vi "Deco meds ME.vi"(5 "Eeprom":T2 {"Analogicas 32"."?" items=["1", "2", "4", "8", "16", "32", "64", "128", "256"]; "Analogicas 32"."?" items=["Lineal"=15, "Cuadrática"=14]; "Analogicas 32"."unsigned byte array[0]" items=["10000", "1000", "100", "10", "8000", "800", "80", "8", "4000", "400", "40", "4", "2000", "200", "20", "2"]; "Analogicas 16"."?" items=["1", "2", "4", "8", "16", "32", "64", "128", "256"]; "Analogicas 16"."?" items=["Lineal"=15, "Cuadrática"=14]; "Analogicas 16"."unsigned byte array[0]" items=["10000", "1000", "100", "10", "8000", "800", "80", "8", "4000", "400", "40", "4", "2000", "200", "20", "2"]}, 6 "data IN":string) -> (3 "Med 568":T1)   [LabVIEW 2010]
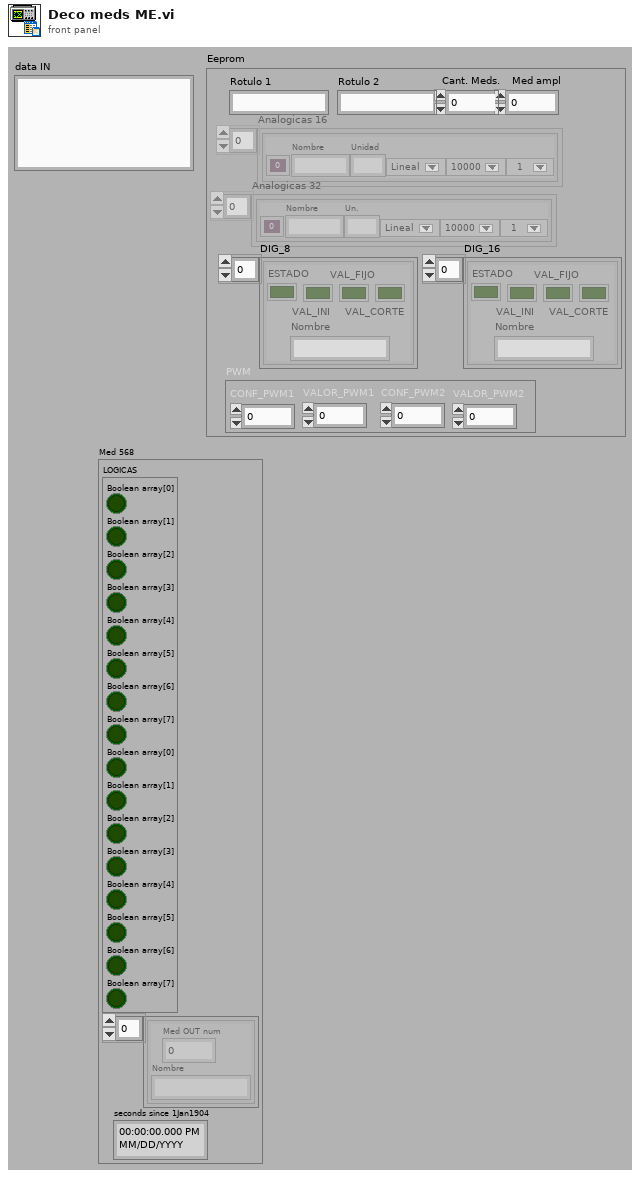
[diagram p1: front panel]
types:
  T1 = cluster{"LOGICAS":cluster{"Boolean array[0]":bool, "Boolean array[1]":bool, "Boolean array[2]":bool, "Boolean array[3]":bool, "Boolean array[4]":bool, "Boolean array[5]":bool, "Boolean array[6]":bool, "Boolean array[7]":bool, "Boolean array[0]":bool, "Boolean array[1]":bool, "Boolean array[2]":bool, "Boolean array[3]":bool, "Boolean array[4]":bool, "Boolean array[5]":bool, "Boolean array[6]":bool, "Boolean array[7]":bool}, cluster{"Med OUT num":dbl, "Nombre":string}[], "seconds since 1Jan1904":timestamp}
  T2 = cluster{"Rotulo 1":string, "Rotulo 2":string, "Cant. Meds.":u8, "Med ampl":u8, "Analogicas 16":cluster{"Nº":i32, "Nombre":string, "Unidad":string, u8, "unsigned byte array[0]":u8, u8}[], "Analogicas 32":cluster{i32, "Nombre":string, "Un.":string, u8, "unsigned byte array[0]":u8, u8}[], "DIG_8":cluster{"ESTADO":bool, "VAL_INI":bool, "VAL_FIJO":bool, "VAL_CORTE":bool, "Nombre":string}[], "DIG_16":cluster{"ESTADO":bool, "VAL_INI":bool, "VAL_FIJO":bool, "VAL_CORTE":bool, "Nombre":string}[], "PWM":cluster{"CONF_PWM1":u8, "VALOR_PWM1":u8, "CONF_PWM2":u8, "VALOR_PWM2":u8}}
  T3 = cluster{"Boolean array[0]":bool, "Boolean array[1]":bool, "Boolean array[2]":bool, "Boolean array[3]":bool, "Boolean array[4]":bool, "Boolean array[5]":bool, "Boolean array[6]":bool, "Boolean array[7]":bool, "Boolean array[0]":bool, "Boolean array[1]":bool, "Boolean array[2]":bool, "Boolean array[3]":bool, "Boolean array[4]":bool, "Boolean array[5]":bool, "Boolean array[6]":bool, "Boolean array[7]":bool}
  T4 = cluster{"Nº":i32, "Nombre":string, "Unidad":string, u8, "unsigned byte array[0]":u8, u8}[]
  T5 = cluster{i32, "Nombre":string, "Un.":string, u8, "unsigned byte array[0]":u8, u8}[]
  T6 = cluster{"Nº":i32, "Nombre":string, "Un.":string, u8, "unsigned byte array[0]":u8, u8}
  T7 = cluster{"LOGICAS":cluster{"Boolean array[0]":bool, "Boolean array[1]":bool, "Boolean array[2]":bool, "Boolean array[3]":bool, "Boolean array[4]":bool, "Boolean array[5]":bool, "Boolean array[6]":bool, "Boolean array[7]":bool, "Boolean array[0]":bool, "Boolean array[1]":bool, "Boolean array[2]":bool, "Boolean array[3]":bool, "Boolean array[4]":bool, "Boolean array[5]":bool, "Boolean array[6]":bool, "Boolean array[7]":bool}, cluster{"Med OUT num":dbl, string}[], "seconds since 1Jan1904":timestamp}
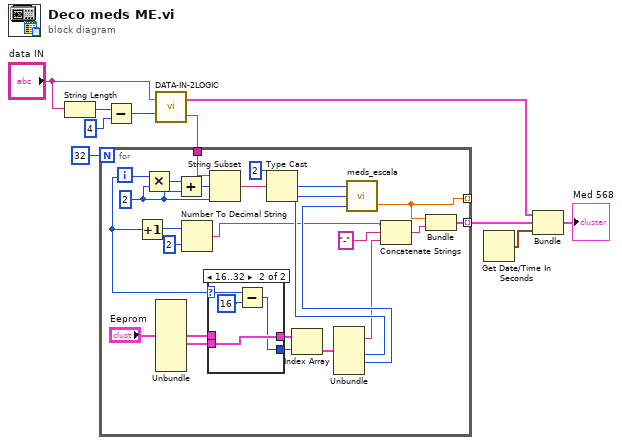
[diagram p0: block diagram]
diagram:
  n1 = String Length(string="data IN") -> (length=w9:i32)
  n2 = Subtract(x=w9, y=4) -> (x-y=w8:i32)
  n3 = call "DATA-IN-2LOGIC.vi"("SIZE"=w8, "data IN"="data IN") -> ("ANALOGICAS"=w5:string, "LOGICAS"=w3:T3)
  n4 = for {
    N: 32 -> [_]
    tunnel: w5 -> [w21]
    tunnel: [w19] -> _ mode=indexing
    tunnel: [w18] -> w2 mode=indexing
    i -> [w17]
    w33 = 2 ("offset (0)")
    n5 = Increment(x=w17) -> (x+1=w16:i32)
    n6 = Multiply(x=w17, y=w33) -> (x*y=w34:i32)
    n7 = Unbundle("Eeprom") -> ("Analogicas 16"=w30:T4, "Analogicas 32"=w29:T5)  [unwired: 7 out]
    n8 = Add(x=w34, y=w33) -> (x+y=w20:i32)
    n9 = Number To Decimal String(number=w16, width (-)=i16 2) -> (decimal integer string=w11:string)
    n10 = case shown="16..32" w17 {
      selector: w17 -> [w35 w40]
      tunnel: w30 -> [w36 _]
      tunnel: w29 -> [_ w38]
      tunnel: [w36 w38] -> w28
      tunnel: [w35 w37] -> w27
      frame 0..15, Default {
      }
      frame 16..32 {
        n11 = Subtract(x=w40, y=16) -> (x-y=w37:i32)
      }
    }
    n12 = String Subset(string=w21, offset (0)=w20, length (rest)=w33) -> (substring=w22:string)
    n13 = Type Cast(type=i16 2 ("length (rest)"), x=w22) -> (*(type *) &x=w23:i16)
    n14 = Index Array(array=w28, index=w27) -> (element=w26:T6)
    n15 = Unbundle(w26) -> ("Nombre"=w13:string, w25:u8, "unsigned byte array[0]"=w24:u8)  [unwired: 3 out]
    n16 = call "meds_escala.vi"("F. Escala"=w24, "linealidad"=w25, "Med IN"=w23) -> ("Med OUT num"=w19:dbl)  [unwired: 1 out]
    n17 = Concatenate Strings(w11, "-", w13) -> (w14:string)
    n18 = Bundle("Med OUT num"=w19, w14) -> (w18:cluster{"Med OUT num":dbl, string})  [unwired: 1 in]
  }
  n19 = Get Date/Time In Seconds() -> (seconds since 1Jan1904=w4:timestamp)
  n20 = Bundle("LOGICAS"=w3, w2, "seconds since 1Jan1904"=w4) -> (→"Med 568":T7)  [unwired: 1 in]
